vi "checkFinishKickPenaltyAllyPlayVSS.vi"(8 "error in (no error)":errorcluster, 9 "last command_interpreted":T1, 10 "Game in":refnum<class "Game.lvclass">, 11 "KickPenaltyAllyPlayVSS in":refnum<class "KickPenaltyAllyPlayVSS.lvclass">) -> (0 "error out":errorcluster, 2 "result":bool, 3 "KickPenaltyAllyPlayVSS out":refnum<class "KickPenaltyAllyPlayVSS.lvclass">)   [LabVIEW 2020, in "KickPenaltyAllyPlayVSS.lvclass"]
uses:
  KickPenaltyAllyPlayVSS.lvclass
  Game_class/Game.lvclass
  Referee_class/command_interpreted.ctl
  Game_class/Game.lvclass/Game.ctl
  Events_class/Events.lvclass/Events.ctl
  Game_class/Read Referee.vi
  Game_class/Read EventsRef.vi
  Events_class/Read ball_out.vi
  Events_class/Read touch.vi
  Events_class/Read ball_out_of_vision.vi
  Events_class/Read id_touch.vi
  Referee_class/Referee.lvclass
  Events_class/Events.lvclass
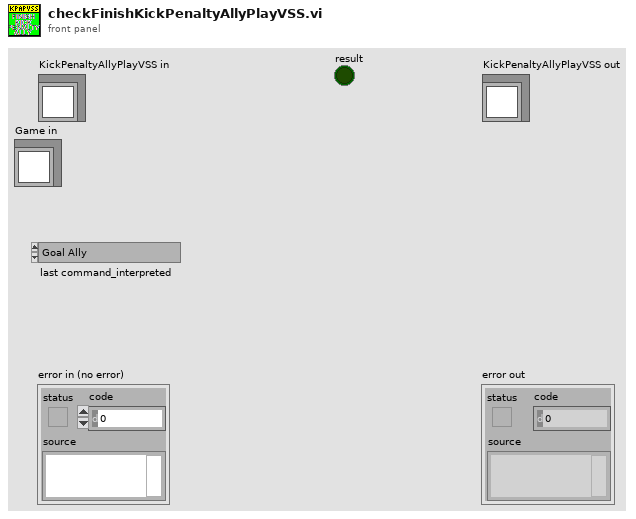
[diagram p1: front panel]
types:
  T1 = typedef "command_interpreted.ctl" = enum16{"Goal Ally", "Goal Enemy", "Ball Placement Enemy", "Ball Placement Ally", "Normal Half Time", "Extra Time  Break", "Extra Half Time", "None", "Post Game", "PKA Normal Start", "Prepare Kickoff Ally", "PKE Normal Start", "Prepare Kickoff Enemy", "Force Start", "Halt", "Timeout", "Prepare Penalty Ally", "Prepare Penalty Enemy", "PPA NormalStart", "PPE Normal Start", "Indirect Free Ally", "Direct Free Enemy", "Direct Free Ally", "Indirect Free Enemy", "Stop"}
  T2 = enum16{"AUTO", "GAME_ON", "STOP", "KICKOFF", "FREE_BALL", "GOAL_KICK", "PENALTY_KICK", "FREE_KICK"}
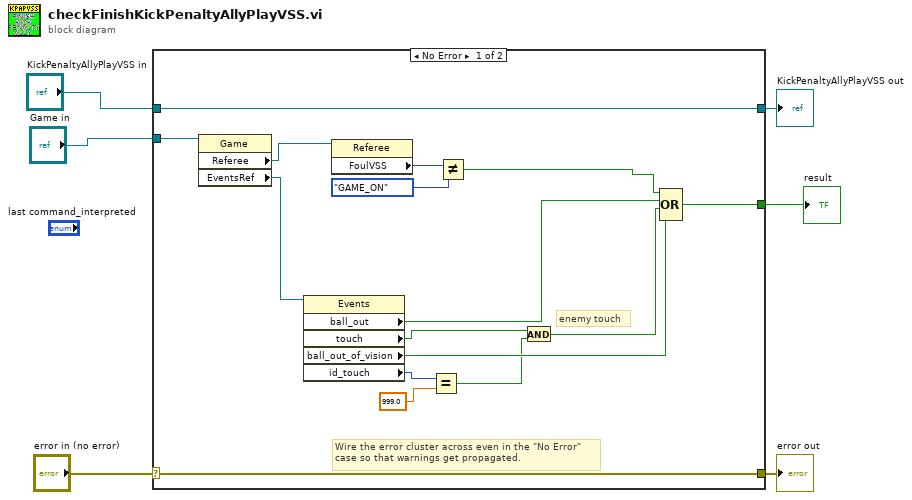
[diagram p0: block diagram]
diagram:
  n1 = case shown="No Error" "error in (no error)" {
    selector: "error in (no error)" -> [w21 w24]
    tunnel: [w21 w24] -> w5
    tunnel: [w22 w23] -> w3
    tunnel: "KickPenaltyAllyPlayVSS in" -> [w22 w23]
    tunnel: [w12 _] -> w2
    tunnel: "Game in" -> [w11 _]
    frame No Error {
      # "enemy touch"
      # "Wire the error cluster across even in the \"No Error\"\ncase so that warnings get propagated."
      n2 = property class="Game"(reference=w11) -> ("Referee"=w7:refnum<class "Referee.lvclass">, "EventsRef"=w20:refnum<class "Events.lvclass">)  [unwired: 1 in, 2 out]
      n3 = property class="Events"(reference=w20) -> ("ball_out"=w19:bool, "touch"=w16:bool, "ball_out_of_vision"=w18:bool, "id_touch"=w15:i32)  [unwired: 1 in, 2 out]
      n4 = property class="Referee"(reference=w7) -> ("FoulVSS"=w10:T2)  [unwired: 1 in, 2 out]
      n5 = Equal?(x=w15, y=999.0) -> (x = y?=w13:bool)
      n6 = Not Equal?(x=w10, y=T2."GAME_ON") -> (x != y?=w8:bool)
      n7 = And(x=w16, y=w13) -> (x .and. y?=w17:bool)
      n8 = Compound Arithmetic op=OR(w8, w19, w17, w18) -> (w12:bool)
    }
    frame Error {
    }
  }
  "error out" <- w5
  "KickPenaltyAllyPlayVSS out" <- w3
  "result" <- w2
